vi "Test Get All with PI.vi"(8 "error out":errorcluster, 11 "Connection Refnum":T1) -> (0 "error out 2":errorcluster, 2 "tests":string[](array[string]), 3 "Connection Refnum 2":T1)   [LabVIEW 2011]
uses:
  SI.LIB/ODBC/SQL Controls/Connection Refnum.ctl
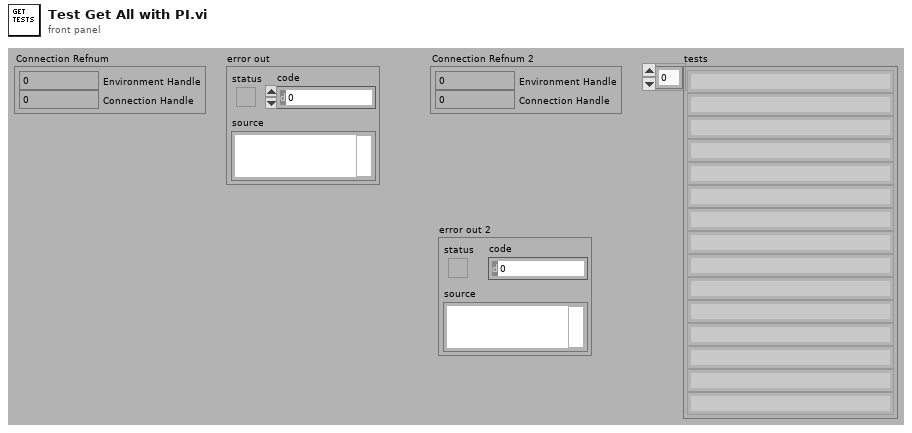
[diagram p1: front panel]
types:
  T1 = typedef "Connection Refnum.ctl" = cluster{"Environment Handle":i32, "Connection Handle":i32}
  T2 = typedef "Field Record.ctl" = cluster{"ixField":i32, "iSequenceOrder":i32, "sxFieldId":string, "sxSequenceId":string, "sDisplayName":string, "sValue":string, "sUnits":string, "nDataType":T3, "nNextItem":T4, "fSystem":bool, "fSystemValue":bool, "fRequired":bool, "fSetAtTest":bool, "fTestField":bool, "fDeleted":bool, "fIndexed":bool, "fFreeList":bool}
  T3 = typedef "Field DataTypes.ctl" = enum32{"text", "numeric", "list", "timestamp", "boolean"}
  T4 = typedef "Field NextItem.ctl" = enum32{"Reset", "Retain", "Auto-Increment"}
  T5 = typedef "Test Record.ctl" = cluster{"ixTest":i32, "sxTestId":string, "sVersion":string, "sDriverTypes":string[], "sDescription":string, "iQuickMode":i32}
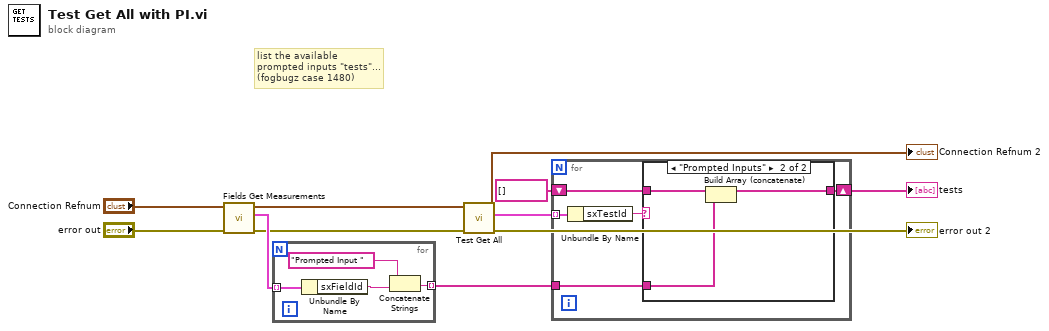
[diagram p0: block diagram]
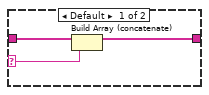
[diagram p2: hidden frame]
diagram:
  # "list the available\nprompted inputs \"tests\"...\n(fogbugz case 1480)"
  n1 = call "Fields Get Measurements.vi"("error in (no error)"="error out", "Connection Refnum"="Connection Refnum") -> ("error out"=w6:errorcluster, "Measurement Fields"=w11:T2[], "dup Connection Refnum"=w7:T1)  [unwired: 1 in, 6 out]
  n2 = for {
    tunnel: w11 -> [w15] mode=indexing
    tunnel: [w12] -> w4 mode=indexing
    n3 = Unbundle By Name(w15) -> ("sxFieldId"=w13:string)
    n4 = Concatenate Strings("Prompted Input " ("y"), w13) -> (w12:string)
  }
  n5 = call "Test Get All.vi"("error in (no error)"=w6, "Connection Refnum"=w7) -> ("error out"=→"error out 2":errorcluster, "Test Records"=w10:T5[], "Connection Refnum"=→"Connection Refnum 2":T1)  [unwired: 2 in, 5 out]
  n6 = for {
    tunnel: w10 -> [w20] mode=indexing
    shift-right: [w17] -> w3
    shift-left: string[] [] ("tests") -> [w18]
    tunnel: w4 -> [w16]
    n7 = Unbundle By Name(w20) -> ("sxTestId"=w19:string)
    n8 = case shown="\"Prompted Inputs\"" w19 {
      selector: w19 -> [w23 _]
      tunnel: w18 -> [w22 w26]
      tunnel: [w21 w25] -> w17
      tunnel: w16 -> [_ w24]
      frame Default {
        n9 = Build Array (concatenate)(w22, w23) -> (w21:string[])
      }
      frame "Prompted Inputs" {
        n10 = Build Array (concatenate)(w26, w24) -> (w25:string[])
      }
    }
  }
  "tests" <- w3
